vi "Send Response.vi"(7 "Close? (T)":bool=TRUE, 8 "error in (no error)":errorcluster, 9 "Stream in":refnum<class "Stream.lvclass">, 11 "Response in":refnum<class "Response.lvclass">) -> (0 "error out":errorcluster, 1 "Stream out":refnum<class "Stream.lvclass">, 3 "Response out":refnum<class "Response.lvclass">)   [LabVIEW 2020, in "HTTP Utils.lvlib" / "Response.lvclass"]
uses:
  Response.lvclass
  <vilib>/IlluminatedG/lv-stream/stream/Stream.lvclass
  Response.lvclass/Response.ctl
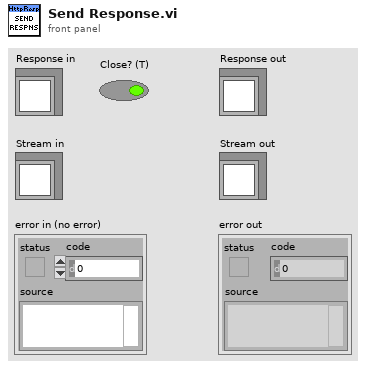
[diagram p1: front panel]
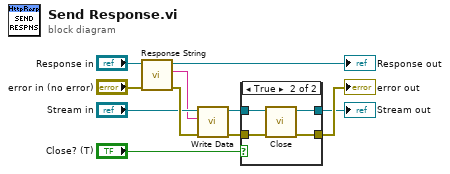
[diagram p0: block diagram]
diagram:
  n1 = call-dynamic "Response String.vi"("error in (no error)"="error in (no error)", "Response in"="Response in") -> ("error out"=w10:errorcluster, "Response String"=w6:string, "Response out"=→"Response out":refnum<class "Response.lvclass">)  [unwired: 7 in]
  n2 = call <vilib>:"Write Data.vi"("error in (no error)"=w10, "Data"=w6, "Stream in"="Stream in") -> ("error out"=w3:errorcluster, "Stream out"=w2:refnum<class "Stream.lvclass">)  [unwired: 7 in]
  n3 = case shown="True" "Close? (T)" {
    tunnel: w3 -> [w12 w16]
    tunnel: w2 -> [w13 w17]
    tunnel: [w13 w15] -> w1
    tunnel: [w12 w14] -> w11
    frame False {
    }
    frame True {
      n4 = call-dynamic "Close.vi"("error in (no error)"=w16, "Stream in"=w17) -> ("error out"=w14:errorcluster, "Stream out"=w15:refnum<class "Stream.lvclass">)  [unwired: 8 in]
    }
  }
  "error out" <- w11
  "Stream out" <- w1
